vi "Start Keepalive HB.vi"(8 "error in (no error)":errorcluster, 11 "WebSocket Connection in":refnum<class "WebSocket Connection.lvclass">) -> (0 "error out":errorcluster, 2 "Keepalive Heartbeat's Enqueuer":refnum<class "Message Enqueuer.lvclass">, 3 "WebSocket Connection out":refnum<class "WebSocket Connection.lvclass">)   [LabVIEW 2021, in "WebSocket Actors.lvlib" / "WebSocket Connection.lvclass"]
uses:
  WebSocket Connection.lvclass
  C:/Program Files/National Instruments/LabVIEW 2021/vi.lib/ActorFramework/Actor/Actor.lvclass
  <vilib>/ActorFramework/Message Enqueuer/Message Enqueuer.lvclass
  WebSocket Connection.lvclass/WebSocket Connection.ctl
  Keepalive Heartbeat/Keepalive Heartbeat.lvclass
  Keepalive Heartbeat/Keepalive Heartbeat.lvclass/Keepalive Heartbeat.ctl
  Keepalive Heartbeat/Write Keepalive.vi
  <vilib>/ActorFramework/Actor/Actor.lvclass
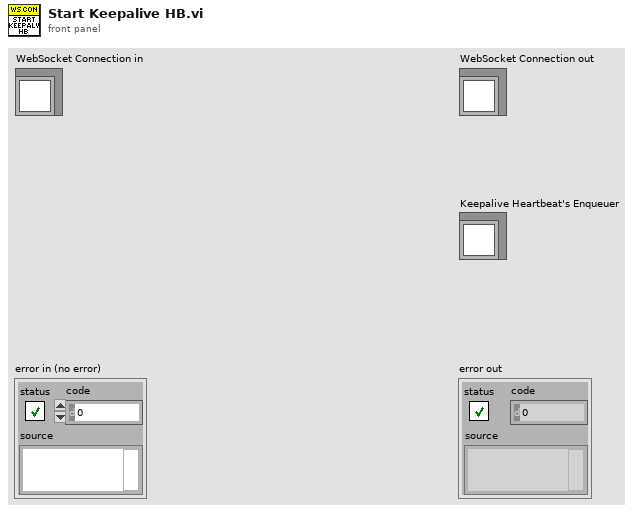
[diagram p1: front panel]
types:
  T1 = typedef "WebSocket Actors.lvlib/WebSocket Connection.lvclass/Keepalive.ctl" = cluster{"Enabled":bool, "Ping Interval (ms)":u32, "Ping Timeout (ms)":u32}
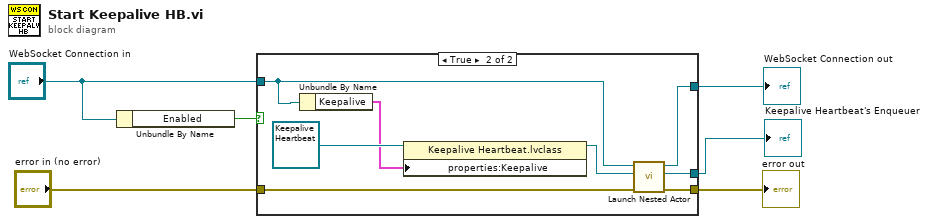
[diagram p0: block diagram]
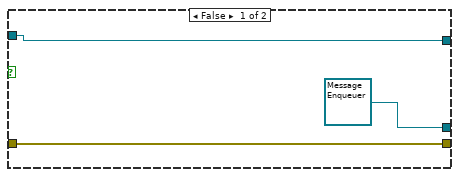
[diagram p2: hidden frame]
diagram:
  n1 = Unbundle By Name("WebSocket Connection in") -> ("Enabled"=w4:bool)
  n2 = case shown="True" w4 {
    tunnel: "error in (no error)" -> [w9 w17]
    tunnel: [w9 w16] -> w5
    tunnel: "WebSocket Connection in" -> [w8 w12]
    tunnel: [w8 w14] -> w2
    tunnel: [refnum<class "Message Enqueuer.lvclass"> refnum ("Nested Actor's Enqueuer") w10] -> w1
    frame False {
    }
    frame True {
      n3 = Unbundle By Name(w12) -> ("Keepalive"=w11:T1)
      n4 = property class="Keepalive Heartbeat.lvclass"(reference=refnum<class "Keepalive Heartbeat.lvclass"> refnum ("WebSocket Actors.lvlib:Keepalive Heartbeat.lvclass"), "properties:Keepalive"=w11) -> (reference out=w13:refnum<class "Keepalive Heartbeat.lvclass">)  [unwired: 1 in, 1 out]
      n5 = call <vilib>:"Launch Nested Actor.vi"("error in (no error)"=w17, "Nested Actor"=w13, "Caller Actor in"=w12) -> ("error out"=w16:errorcluster, "Nested Actor's Enqueuer"=w10:refnum<class "Message Enqueuer.lvclass">, "Caller Actor out"=w14:refnum<class "WebSocket Connection.lvclass">)  [unwired: 6 in]
    }
  }
  "error out" <- w5
  "WebSocket Connection out" <- w2
  "Keepalive Heartbeat's Enqueuer" <- w1
